vi "Apply Relay State.vi"(8 "error in":errorcluster, 9 "State":bool, 10 "Name":string, 11 "SwitchMatrix in":refnum<class "SwitchMatrix.lvclass">) -> (0 "error out":errorcluster, 3 "SwitchMatrix out":refnum<class "SwitchMatrix.lvclass">)   [LabVIEW 2019, in "SwitchMatrix.lvlib" / "SwitchMatrix.lvclass"]
uses:
  Library/SwitchMatrix.lvclass
  Library/SwitchMatrix.lvclass/SwitchMatrix.ctl
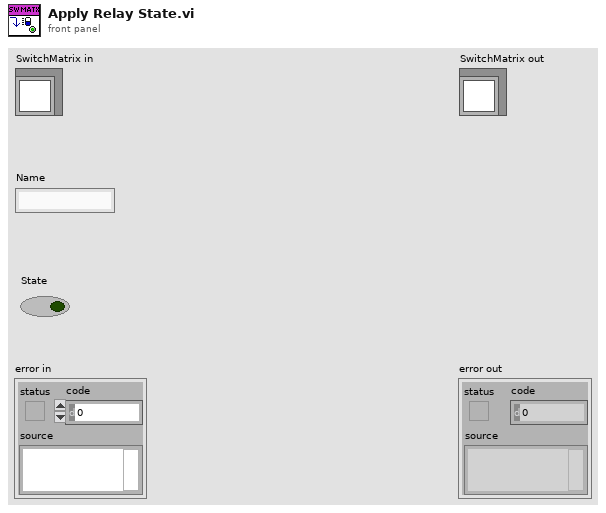
[diagram p1: front panel]
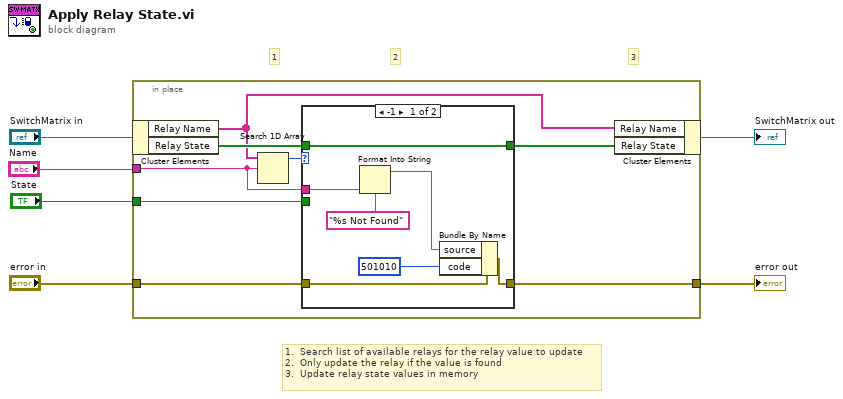
[diagram p0: block diagram]
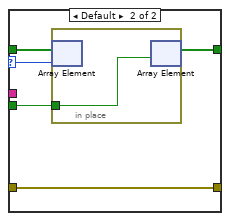
[diagram p2: hidden frame]
diagram:
  # "3"
  # "2"
  # "1"
  # "1.  Search list of available relays for the relay value to update\n2.  Only update the relay if the value is found\n3.  Update relay state values in memory"
  n1 = in-place {
    in-place-border: "error in" -> [w9]
    in-place-border: [w8] -> w1
    in-place-border: "Name" -> [w7]
    in-place-border: "State" -> [w13]
    n2 = in-place-cluster #1("SwitchMatrix in") -> ("Relay Name"=w10:string[], "Relay State"=w14:bool[])
    n3 = Search 1D Array(1D array=w10, element=w7) -> (index of element=w11:i32)  [unwired: 1 in]
    n4 = case shown="-1" w11 {
      selector: w11 -> [_ w23]
      tunnel: w14 -> [w21 w26]
      tunnel: w13 -> [_ w25]
      tunnel: [w21 w24] -> w12
      tunnel: w9 -> [w20 w22]
      tunnel: [w19 w22] -> w8
      tunnel: w7 -> [w17 _]
      frame -1 {
        n5 = Format Into String(format string="%s Not Found", w17) -> (resulting string=w15:string)  [unwired: 2 in, 1 out]
        n6 = Bundle By Name(cluster=w20, "source"=w15, "code"=501010) -> (w19:errorcluster)
      }
      frame Default {
        n7 = in-place {
          in-place-border: w25 -> [w27]
          n8 = in-place-array #2(w26, w23) -> ()  [unwired: 1 out]
          n9 = in-place-array #2(w27) -> (w24:bool[])  [unwired: 1 out]
        }
      }
    }
    n10 = in-place-cluster #1("Relay Name"=w10, "Relay State"=w12) -> (→"SwitchMatrix out":refnum<class "SwitchMatrix.lvclass">)
  }
  "error out" <- w1
